vi "Build Endpoint.vi"(8 "error in (no error)":errorcluster, 9 "Port":u16, 10 "Address":string, 11 "RemoteControl.ZMQ in":refnum<class "RemoteControl.ZMQ.lvclass">) -> (0 "error out":errorcluster, 3 "RemoteControl.ZMQ out":refnum<class "RemoteControl.ZMQ.lvclass">)   [LabVIEW 2019, in "RemoteControl.ZMQ.lvclass"]
uses:
  RemoteControl.ZMQ.lvclass
  RemoteControl.ZMQ.lvclass/RemoteControl.ZMQ.ctl
  <vilib>/addons/zeromq/zeromq.lvlib
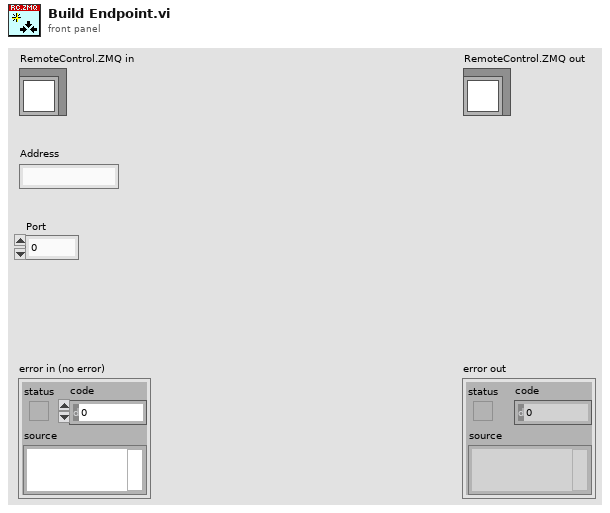
[diagram p1: front panel]
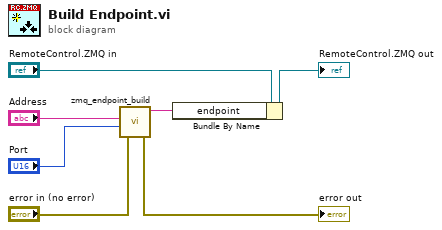
[diagram p0: block diagram]
diagram:
  n1 = call <vilib>:"zmq_endpoint_build.vi"("error in"="error in (no error)", "port"="Port", "address"="Address") -> ("error out"=→"error out":errorcluster, "endpoint"=w1:string)  [unwired: 2 in, 1 out]
  n2 = Bundle By Name(cluster="RemoteControl.ZMQ in", "endpoint"=w1) -> (→"RemoteControl.ZMQ out":refnum<class "RemoteControl.ZMQ.lvclass">)
